vi "RS_wrapper.vi"(11 "Cluster":cluster{i32, i32, i32, bool, string, string}={0, 0, 0, TRUE, "", ""}) -> ()   [LabVIEW 2019, in "Protocols.lvlib"]
uses:
  Protocols.lvlib
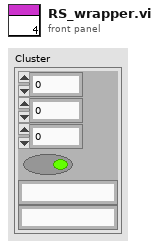
[diagram p1: front panel]
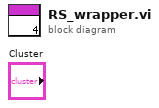
[diagram p0: block diagram]
diagram:
